vi "auto_alignment-v3.vi"(3 "NM-params":T1={"alpha"=1.0, "gamma"=2.0, "rho"=0.5, "sigma"=0.5, "simplex L"=0.5}) -> (1 "xStart":dbl=264.0 format="%#_13g", 2 "yStart":dbl=123.0 format="%#_13g", 4 "Optimized Location":dbl[](array[numeric]), 8 "std dev of simplex values":dbl, 14 "run time (s)":dbl)   [LabVIEW 2024]
uses:
  <vilib>/Math Plots/3D Math Plots/3D Contour/3D Contour XCtrl/3D Contour.xctl
  208f4aca-97d4-4ce0-8583-53fc1167a3ec.vi
  <vilib>/numeric/Random Number (Range) DBL.vi
  2150a5ec-3bbc-4184-8c90-cd07ede4a1ff.vi
  5b59031f-b1ff-41af-80a7-e72a33ebffa1.vi
  <vilib>/Analysis/baseanly.llb/Real Dot Product.vi
  <vilib>/Array/Sort 2D Array - Pop Stack.vi
  <vilib>/Array/Sort 2D Array - Push Stack.vi
  5b59031f-b1ff-41af-80a7-e72a33ebffa1.vi/269d4b3b-47f5-49e3-8884-44851e4dd9d5.vi
  5b59031f-b1ff-41af-80a7-e72a33ebffa1.vi/6d99389c-673d-4efb-bf33-19b32bcf4cf8.vi
  <vilib>/Utility/file.llb/Read Delimited Spreadsheet (string).vi
  <vilib>/gmath/interp.llb/Create Mesh Grid (2D) (x,y arrays).vi
  <vilib>/Math Plots/3D Math Plots/3D Contour/3D Contour Datatype/Public/Plot Helper (Matrix).vi
  <vilib>/Utility/file.llb/Write Delimited Spreadsheet (DBL).vi
  <vilib>/Analysis/NI_AALBase.lvlib
  O:/DSG/Tyler/EIC/DIRC/daq/automated/Thorlabs.MotionControl.IntegratedStepperMotorsCLI.dll
  Thorlabs.MotionControl.IntegratedStepperMotorsCLI.dll
  <vilib>/Analysis/NI_AALPro.lvlib
  <vilib>/Math Plots/3D Math Plots/3D Contour/3D Contour Datatype/3D Contour Datatype.lvclass
  <vilib>/gmath/NI_Gmath.lvlib
panel:
  out "3D Contour":refnum<class "3D Plot Datatype.lvclass">[](xcontrol)
  out "z-angle converge":bool
  in  "z-angle-limit":dbl=0.04 caption="Z-Angle Convergence Goal"
  in  "squError-limit":dbl=0.04 caption="Squared Error Convergence Goal"
  out "angle-to-z":dbl
  out "squared error limit":bool
  out "SquError":dbl
  out "x_c":dbl[](array[numeric])
  out "x_e":dbl[](array[numeric])
  out "x_r":dbl[](array[numeric])
  out "x_o":dbl[](array[numeric])
  out "sim-pdx":dbl[](array[numeric])
  out "sim-pdy":dbl[](array[numeric])
  out "sim-iCorr":dbl[](array[numeric])
  out "sim_max":dbl[](array[numeric])
  out "sim_x-range":dbl[](array[numeric])
  out "sim_y-range":dbl[](array[numeric])
  out "termination-test-simplex":dbl[][](array[numeric])
  out "timeout":bool
  out "simplex converge":bool
  out "value converge":bool
  out "simplex leg lengths":dbl[](array[numeric])
  out "nPts tested":dbl
  out "sim-data":dbl[][](array[numeric])
  in  "simplex-limit":dbl=1e-06 caption="Simplex Length Convergence Goal" format="%#_13g"
  in  "value-limit":dbl=1e-06 caption="Value Convergence Goal" format="%#_13g"
  out "Pts Tested":dbl[][](array[numeric])
  in  "stop":bool
  # "Test Sub-Points"
  # "centroid"
  # "reflection point"
  # "expansion point"
  # "contraction point"
  # "Model Data"
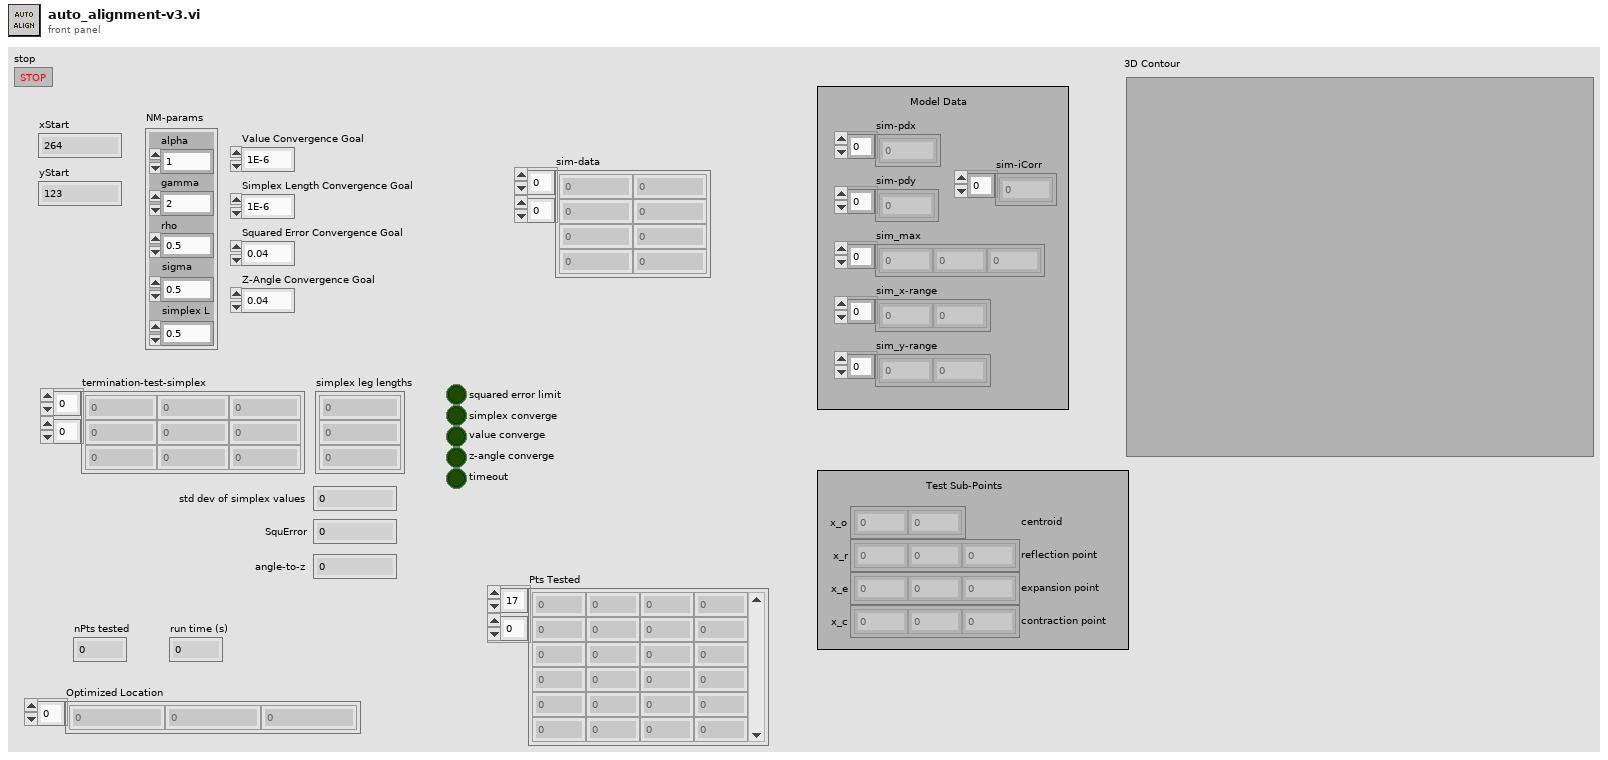
[diagram p1: front panel]
types:
  T1 = cluster{"alpha":dbl, "gamma":dbl, "rho":dbl, "sigma":dbl, "simplex L":dbl}
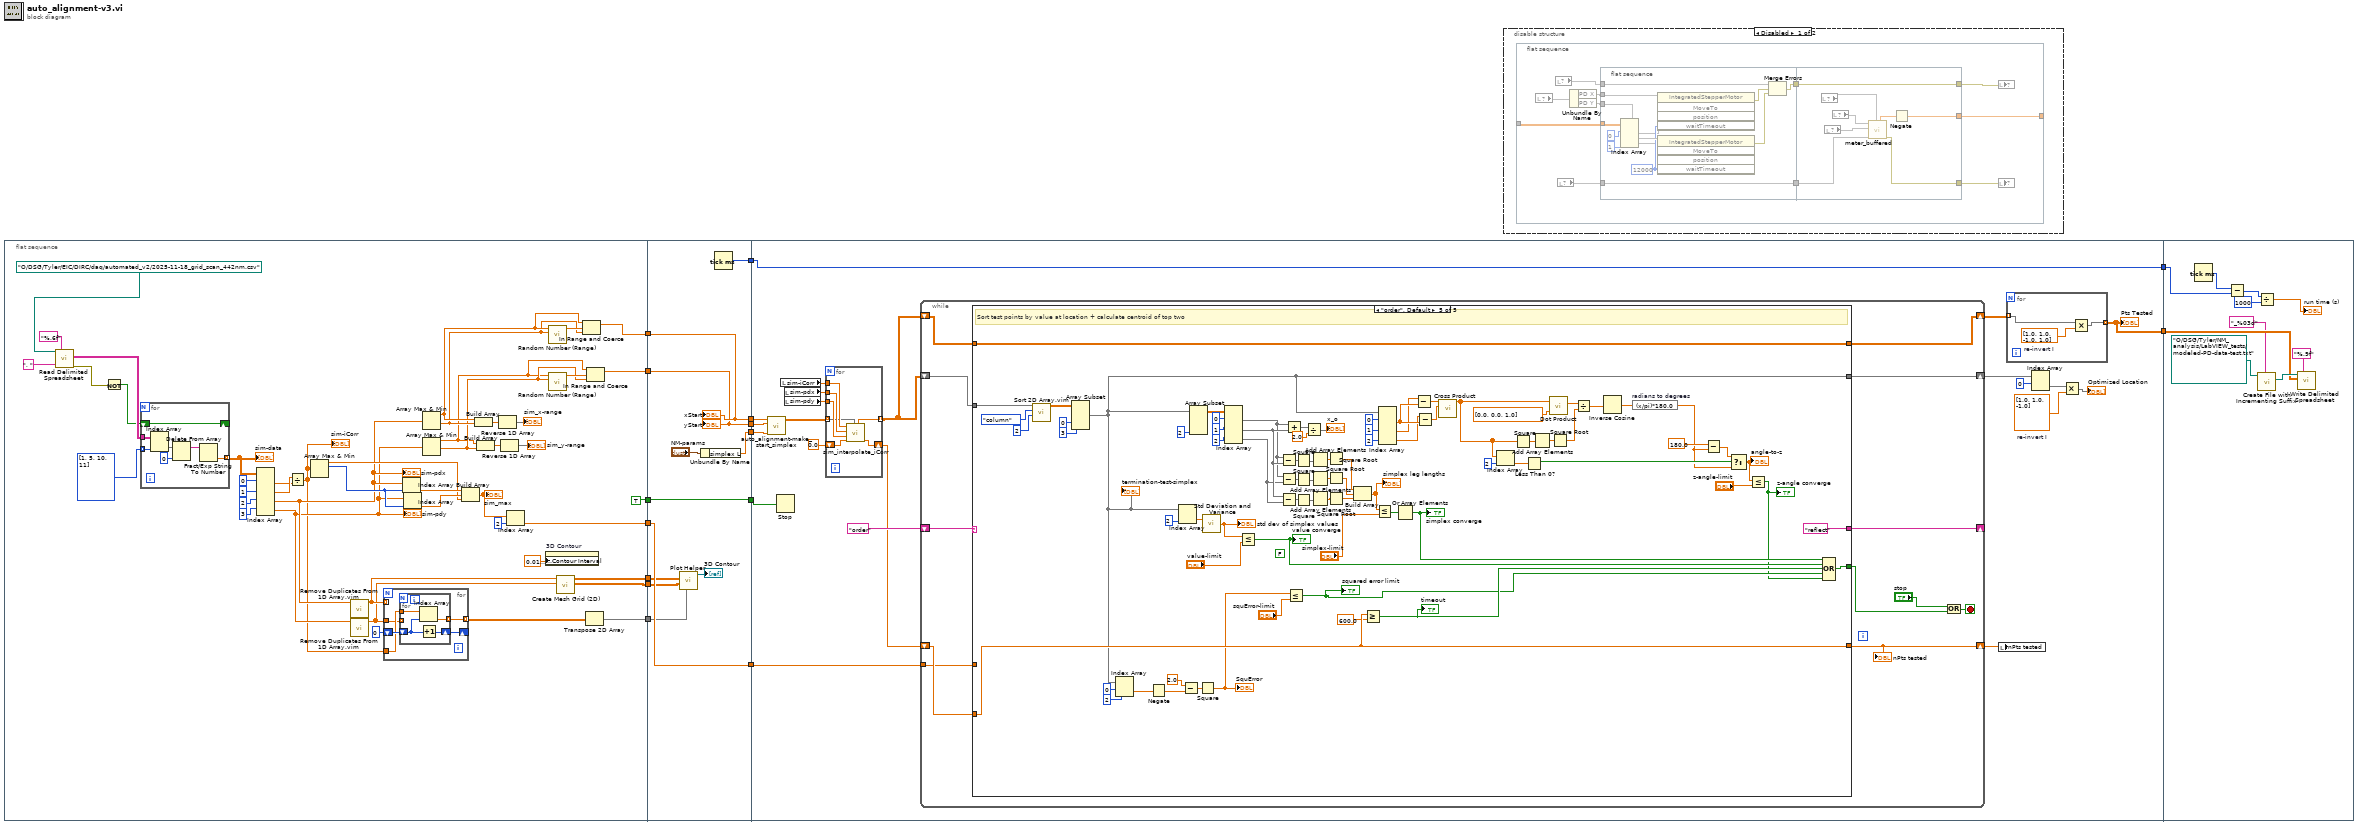
[diagram p0: block diagram]
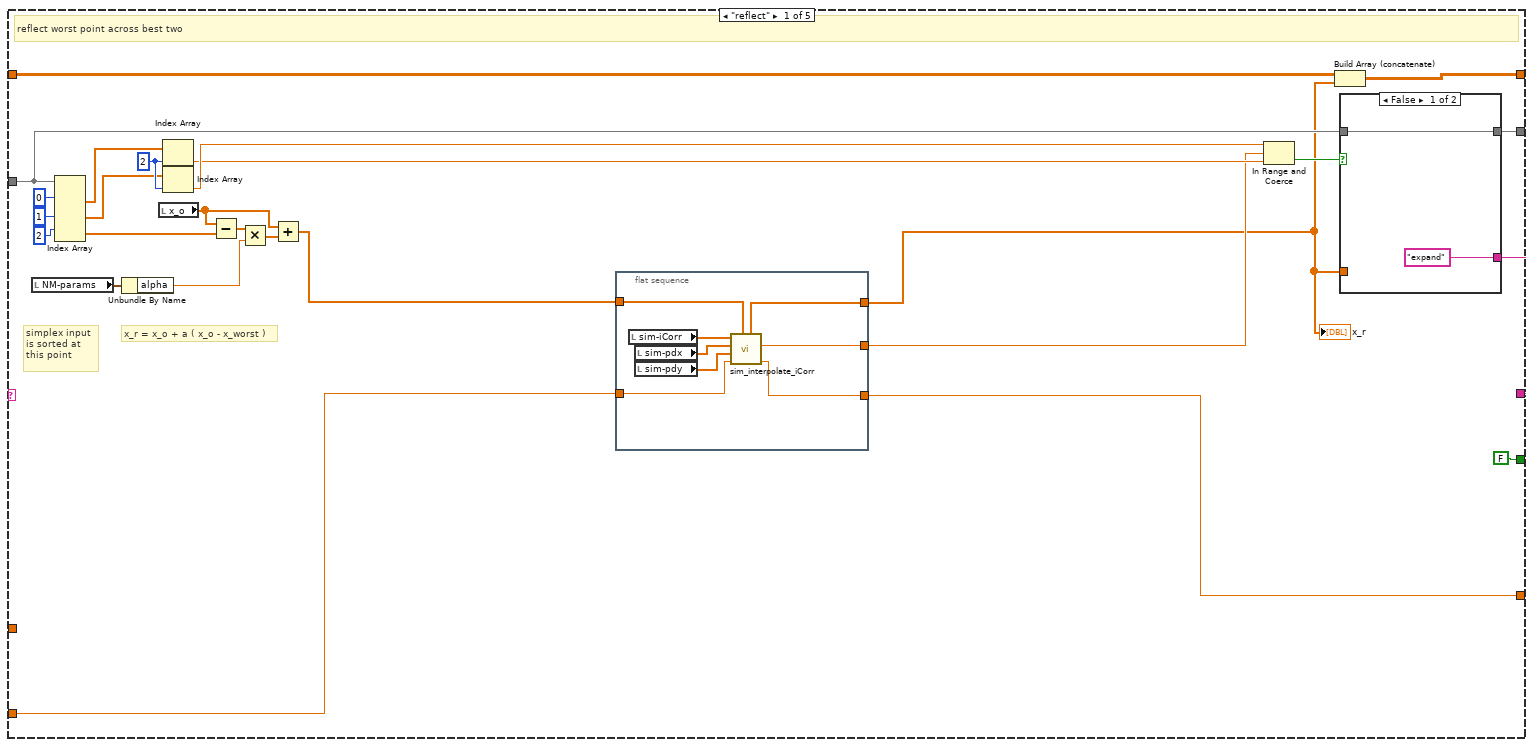
[diagram p3: hidden frame]
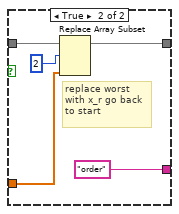
[diagram p4: hidden frame]
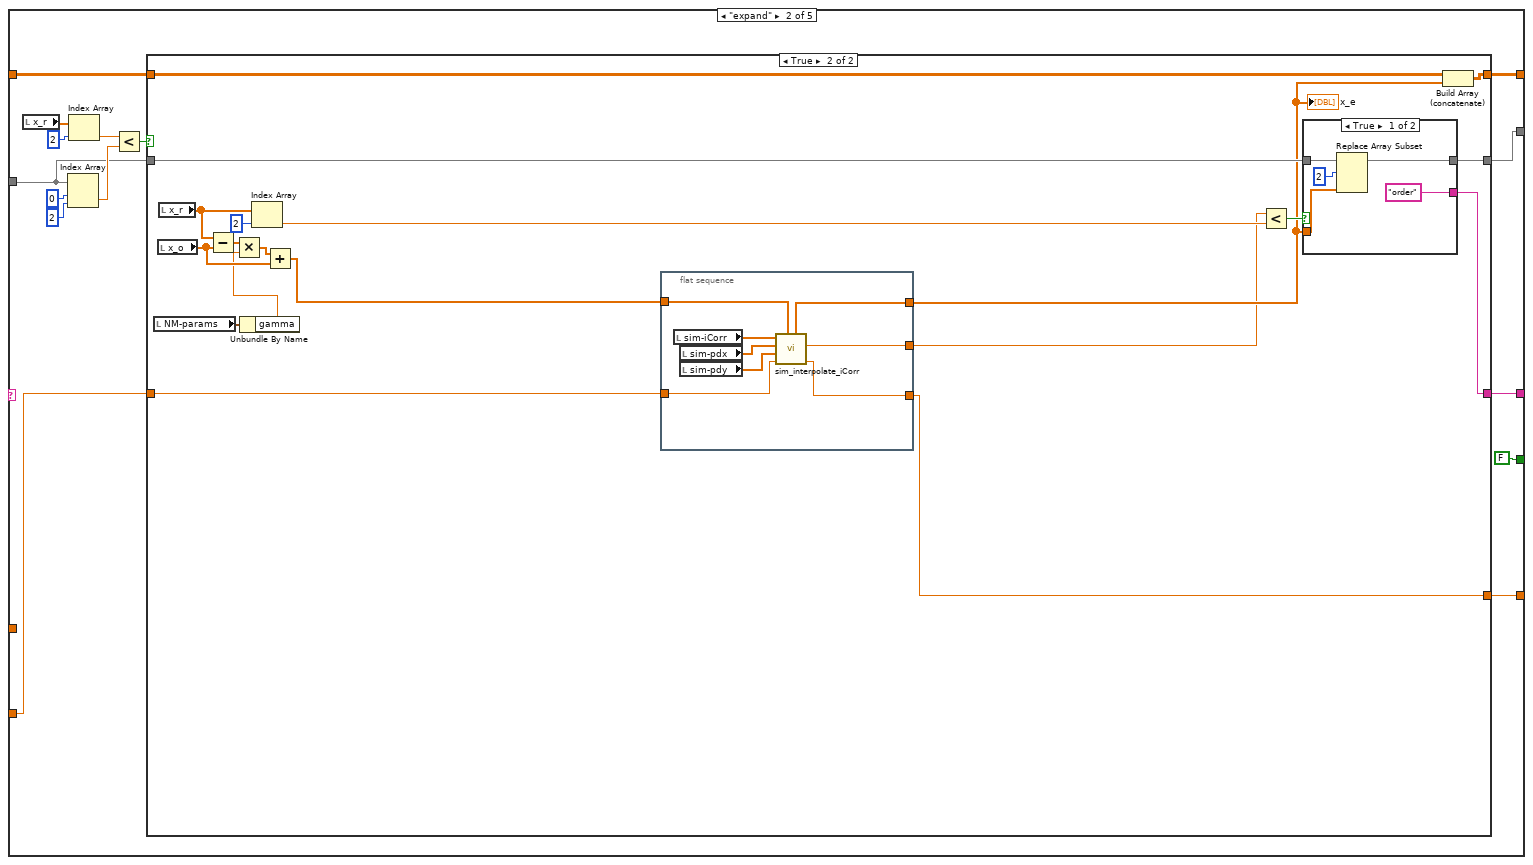
[diagram p5: hidden frame]
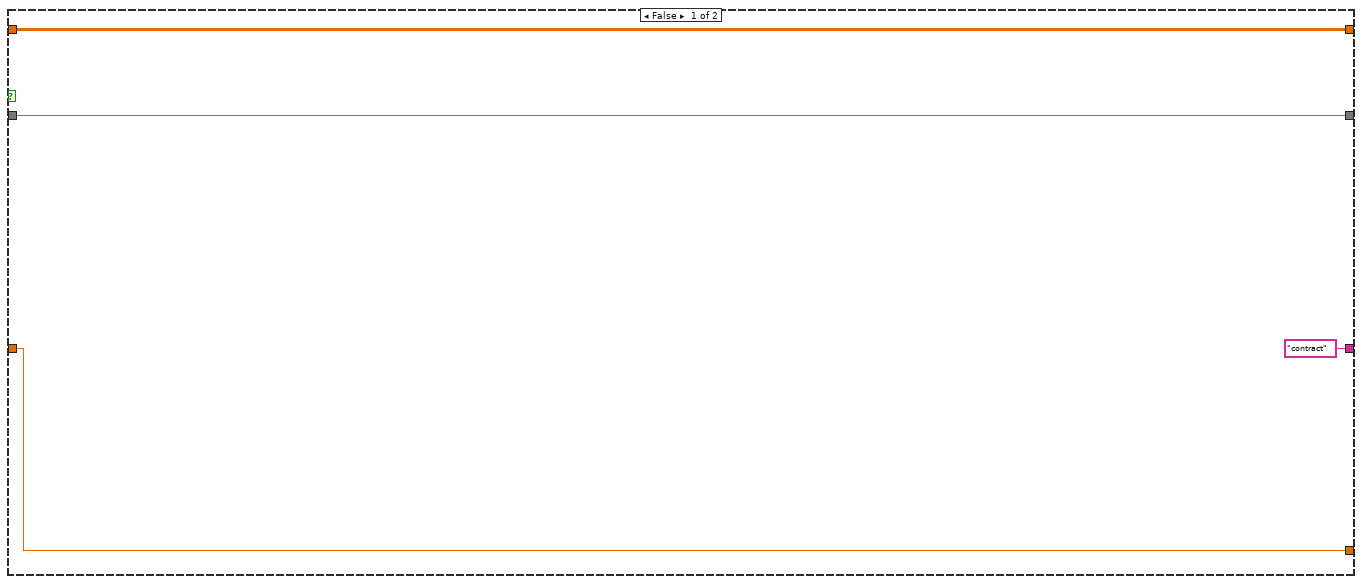
[diagram p6: hidden frame]
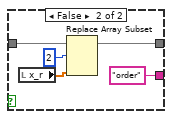
[diagram p7: hidden frame]
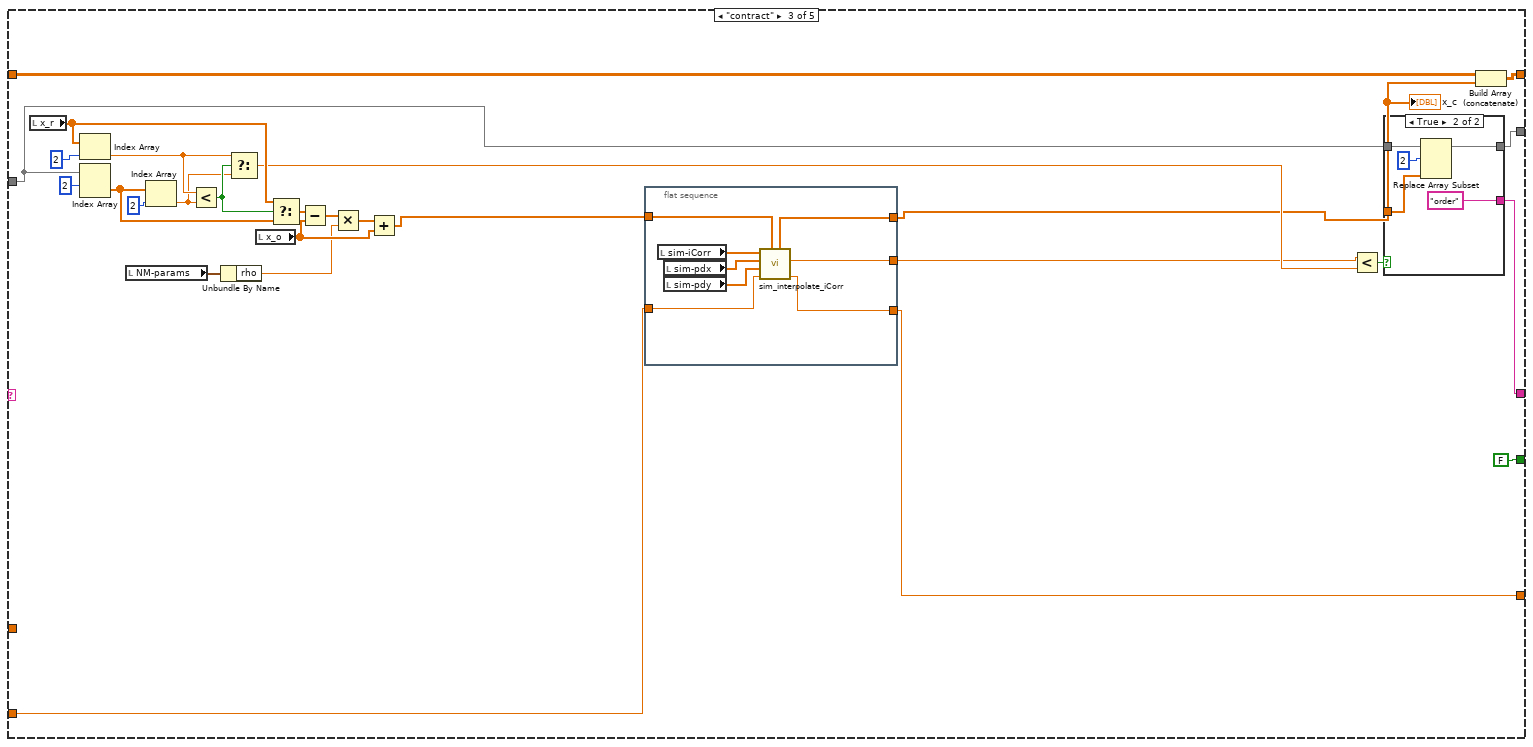
[diagram p8: hidden frame]
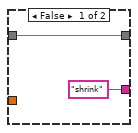
[diagram p9: hidden frame]
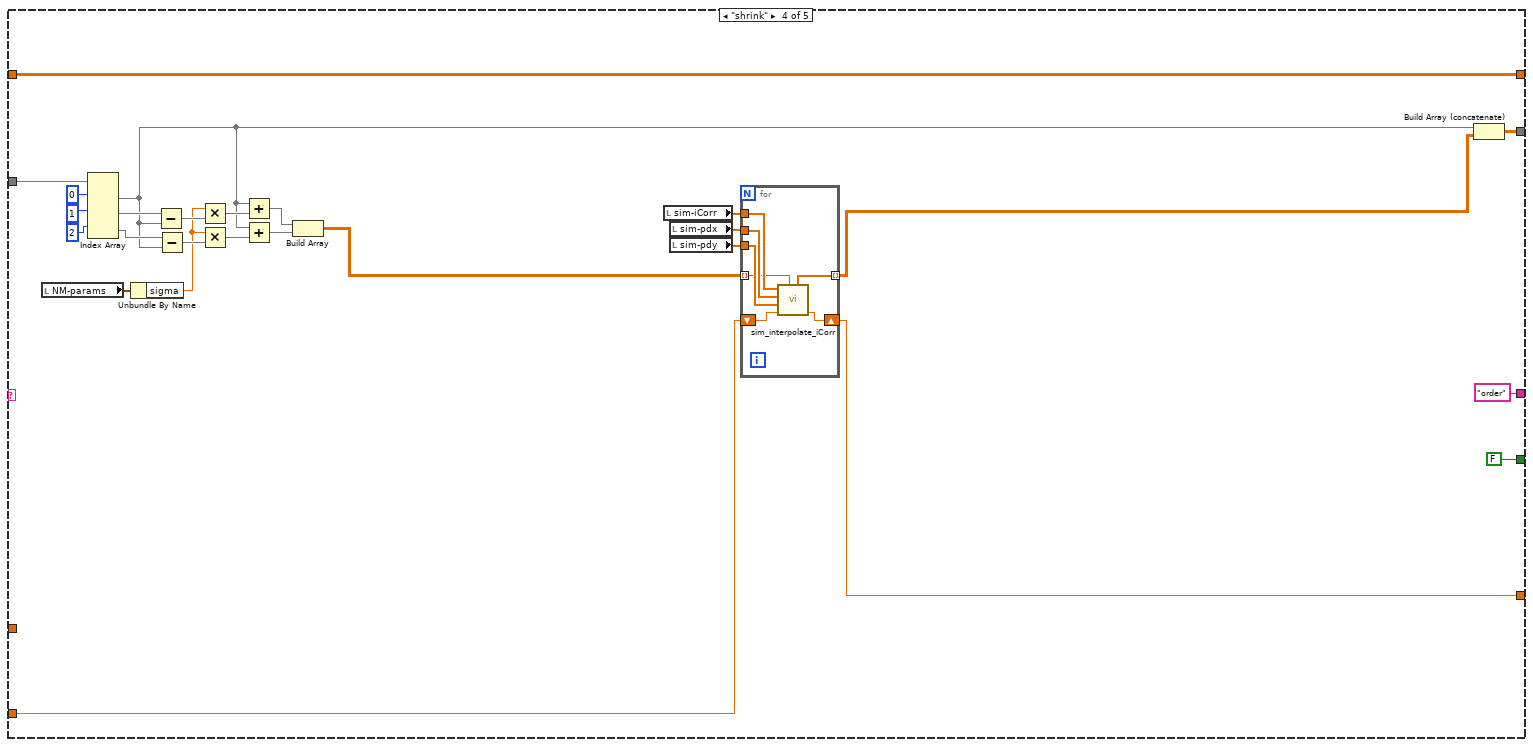
[diagram p10: hidden frame]
diagram:
  n1 = flat-sequence {
    tunnel: [w39] -> w9
    tunnel: [w36] -> w8
    tunnel: [w29] -> w7
    tunnel: [TRUE] -> w5
    tunnel: [w18] -> w3
    tunnel: [w17] -> w2
    tunnel: [w21] -> w1
    tunnel: [w87] -> w15
    tunnel: [w83] -> w13
    tunnel: [w84] -> w12
    tunnel: [w85] -> w11
    tunnel: w9 -> [w84]
    tunnel: w8 -> [w83]
    tunnel: w7 -> [w82]
    tunnel: [w82] -> w6
    tunnel: w5 -> [w81]
    tunnel: [w81] -> w4
    tunnel: w3 -> [w79]
    tunnel: w2 -> [w78]
    tunnel: w1 -> [w77]
    tunnel: w15 -> [w108]
    tunnel: [w108] -> w14
    tunnel: w13 -> [w96]
    tunnel: w12 -> [w97]
    tunnel: w11 -> [w95]
    tunnel: [w90] -> w10
    tunnel: w6 -> [w89]
    tunnel: w4 -> [w88]
    tunnel: w14 -> [w391]
    tunnel: w10 -> [w386]
    frame #0 {
      n2 = call-poly <vilib>:"Read Delimited Spreadsheet.vi"("file path (dialog if empty)"=path "O:/DSG/Tyler/EIC/DIRC/daq/automated_v2/2025-11-18_grid_scan_442nm.csv", "format (%s)"="%.6f" ("format (%.3f)"), "delimiter (\\t)"=", " ("delimiter (\\t)")) -> ("all rows"=w57:string[][], "error out"=w59:errorcluster)  [unwired: 7 in, 4 out]
      n3 = Not(x=w59) -> (.not. x?=w55:bool)
      n4 = for {
        tunnel: i32[] [1, 5, 10, 11] -> [w75] mode=indexing
        tunnel: w57 -> [w76]
        shift-right: [w74] -> _
        shift-left: w55 -> [w74]
        tunnel: [w70] -> w48 mode=indexing
        n5 = Index Array(array=w76, index (col)=w75) -> (element=w73:string[])  [unwired: 1 in]
        n6 = Delete From Array(array=w73, index=0) -> (array with subset deleted=w71:string[])  [unwired: 1 in, 1 out]
        n7 = Fract/Exp String To Number(string=w71) -> (number=w70:dbl[])  [unwired: 3 in, 1 out]
      }
      "sim-data" <- w48
      n8 = Index Array(array=w48, index (row) #1=0 ("index"), index (row) #2=1 ("index (row)"), index (row) #3=2 ("index (row)"), index (row) #4=3 ("index (row)")) -> (element #1=w49:dbl[], element #2=w50:dbl[], element #3=w25:dbl[], element #4=w24:dbl[])  [unwired: 4 in]
      "sim-pdx" <- w25
      "sim-pdy" <- w24
      n9 = Divide(x=w50, y=w49) -> (x/y=w23:dbl[])
      "sim-iCorr" <- w23
      n10 = Array Max & Min(array=w23) -> (max value=w26:dbl, max index (indices)=w47:i32)  [unwired: 2 out]
      n11 = call "Remove Duplicates From 1D Array.vim"("array"=w25) -> ("array with duplicates removed"=w20:dbl[])  [unwired: 10 in]
      n12 = call "Remove Duplicates From 1D Array.vim"("array"=w24) -> ("array with duplicates removed"=w19:dbl[])  [unwired: 10 in]
      n13 = for {
        tunnel: w20 -> [_] mode=indexing
        tunnel: w19 -> [w61]
        tunnel: w23 -> [w62]
        tunnel: [w65] -> w22 mode=indexing
        shift-right: [w63] -> _
        shift-left: 0 -> [w64]
        n14 = for {
          tunnel: [w69] -> w65 mode=indexing
          shift-right: [w68] -> w63
          shift-left: w64 -> [w67]
          tunnel: w62 -> [w66]
          tunnel: w61 -> [_] mode=indexing
          n15 = Index Array(array=w66, index=w67) -> (element=w69:dbl)
          n16 = Increment(x=w67) -> (x+1=w68:i32)
        }
      }
      n17 = Index Array(array=w25, index=w47) -> (element=w46:dbl)
      n18 = Index Array(array=w24, index=w47) -> (element=w45:dbl)
      n19 = Array Max & Min(array=w25) -> (max value=w38:dbl, min value=w37:dbl)  [unwired: 2 out]
      n20 = Array Max & Min(array=w24) -> (max value=w33:dbl, min value=w34:dbl)  [unwired: 2 out]
      n21 = Build Array(w46, w45, w26) -> (w31:dbl[])
      "sim_max" <- w31
      n22 = Build Array(w38, w37) -> (w43:dbl[])
      n23 = Build Array(w33, w34) -> (w44:dbl[])
      n24 = Reverse 1D Array(array=w43) -> (reversed array=→"sim_x-range":dbl[])
      n25 = Reverse 1D Array(array=w44) -> (reversed array=→"sim_y-range":dbl[])
      n26 = Index Array(array=w31, index=2) -> (element=w29:dbl)
      n27 = property on="3D Contour" class="3D Contour (strict)"("Plot Specific:Contour Interval"=sgl 0.02 ("Plot Specific:Contour:Contour Interval")) -> ()  [unwired: 2 in, 2 out]
      n28 = call-poly <vilib>:"Random Number (Range).vi"("lower bound (0)"=w37, "upper bound (100)"=w38) -> ("number"=w40:dbl)  [unwired: 9 in]
      n29 = call-poly <vilib>:"Random Number (Range).vi"("lower bound (0)"=w34, "upper bound (100)"=w33) -> ("number"=w35:dbl)  [unwired: 9 in]
      n30 = call-poly <vilib>:"Create Mesh Grid (2D).vi"("y domain"=w19, "x domain"=w20) -> ("Y"=w17:dbl[][], "X"=w18:dbl[][])  [unwired: 7 in, 1 out]
      n31 = In Range and Coerce(upper limit=w38, x=w40, lower limit=w37) -> (coerced(x)=w39:dbl)  [unwired: 1 out]
      n32 = Transpose 2D Array(2D array=w22) -> (transposed array=w21:dbl[][])
      n33 = In Range and Coerce(upper limit=w33, x=w35, lower limit=w34) -> (coerced(x)=w36:dbl)  [unwired: 1 out]
    }
    frame #1 {
      n34 = call-poly <vilib>:"Plot Helper.vi"("z matrix"=w77, "y matrix"=w78, "x matrix"=w79) -> ("3D Plot lvclass Array out"=→"3D Contour":refnum<class "3D Plot Datatype.lvclass">[])  [unwired: 3 in, 5 out]
      n35 = Unbundle By Name("NM-params") -> ("simplex L"=w85:dbl)
      n36 = Tick Count (ms)() -> (millisecond timer value=w87:u32)
      "xStart" <- w84
      "yStart" <- w83
    }
    frame #2 {
      w103 = dbl[] [1.0, 1.0, -1.0]  # re-invert I
      n37 = call "auto_alignment-make_start_simplex.vi"("L"=w95, "yStart"=w96, "xStart"=w97) -> ("Array"=w98:dbl[][])  [unwired: 8 in]
      n38 = Stop(stop? (T)=w88) -> ()
      n39 = local read "sim-iCorr"() -> (w100:dbl[])
      n40 = local read "sim-pdx"() -> (w102:dbl[])
      n41 = local read "sim-pdy"() -> (w101:dbl[])
      n42 = for {
        shift-right: [w114] -> w93
        shift-left: 0.0 -> [w113]
        tunnel: w98 -> [w116] mode=indexing
        tunnel: [w115] -> w94 mode=indexing
        tunnel: w100 -> [w119]
        tunnel: w101 -> [w117]
        tunnel: w102 -> [w118]
        n43 = call "sim_interpolate_iCorr.vi"("point in"=w116, "nPts in"=w113, "sim-pdy"=w117, "sim-pdx"=w118, "sim-iCorr"=w119) -> ("nPts out"=w114:dbl, "measured-point out"=w115:dbl[])  [unwired: 4 in, 1 out]
      }
      n44 = while {
        shift-right: [w129] -> w107
        shift-left: w94 -> [w128]
        shift-right: [w130] -> _
        shift-left: "order" -> [w131]
        shift-right: [w126] -> w91
        shift-left: w94 -> [w127]
        shift-right: [w121] -> w92
        shift-left: w93 -> [w122]
        tunnel: w89 -> [w120]
        stop <- w123 stop-if-true
        n45 = case shown="\"order\", Default" w131 {
          tunnel: w128 -> [w143 w180 w242 w295 w348]
          tunnel: [FALSE FALSE FALSE FALSE w355] -> w125
          tunnel: [w142 w179 w243 w284 w326] -> w129
          tunnel: [w144 w178 w244 "order" "reflect"] -> w130
          tunnel: w127 -> [w140 w176 w238 w282 w352]
          tunnel: [w139 w175 w237 w282 w352] -> w126
          tunnel: w122 -> [w135 w174 w230 w274 w346]
          tunnel: [w134 w173 w229 w273 w346] -> w121
          tunnel: w120 -> [_ _ _ _ _]
          frame "reflect" {
            w151 = 2 ("index")
            # "simplex input\nis sorted at\nthis point"
            # "x_r = x_o + a ( x_o - x_worst )"
            # "reflect worst point across best two"
            n46 = local read "NM-params"() -> (w138:T1)
            n47 = Index Array(array=w143, index (row) #1=0 ("index (row)"), index (row) #2=1 ("index (row)"), index (row) #3=2 ("index (row)")) -> (element #1=w150:dbl[], element #2=w149:dbl[], element #3=w152:dbl[])  [unwired: 3 in]
            n48 = Unbundle By Name(w138) -> ("alpha"=w137:dbl)
            n49 = local read "x_o"() -> (w145:dbl[])
            n50 = Index Array(array=w150, index=w151) -> (element=w147:dbl)
            n51 = Index Array(array=w149, index=w151) -> (element=w148:dbl)
            n52 = Subtract(x=w145, y=w152) -> (x-y=w156:dbl[])
            n53 = Multiply(x=w156, y=w137) -> (x*y=w155:dbl[])
            n54 = Add(x=w145, y=w155) -> (x+y=w133:dbl[])
            n55 = flat-sequence {
              tunnel: w133 -> [w162]
              tunnel: w135 -> [w161]
              tunnel: [w160] -> w134
              tunnel: [w159] -> w132
              tunnel: [w158] -> w136
              frame #0 {
                n56 = local read "sim-iCorr"() -> (w163:dbl[])
                n57 = local read "sim-pdx"() -> (w164:dbl[])
                n58 = local read "sim-pdy"() -> (w165:dbl[])
                n59 = call "sim_interpolate_iCorr.vi"("point in"=w162, "nPts in"=w161, "sim-pdy"=w165, "sim-pdx"=w164, "sim-iCorr"=w163) -> ("nPts out"=w160:dbl, "iCorr out"=w158:dbl, "measured-point out"=w159:dbl[])  [unwired: 4 in]
              }
            }
            n60 = In Range and Coerce(upper limit=w148, x=w136, lower limit=w147) -> (In Range?=w146:bool)  [unwired: 1 out]
            n61 = Build Array (concatenate)(w140, w132) -> (w139:dbl[][])
            n62 = case shown="False" w146 {
              tunnel: ["expand" "order"] -> w144
              tunnel: w143 -> [w166 w172]
              tunnel: [w166 w169] -> w142
              tunnel: w132 -> [_ w170]
              frame False {
              }
              frame True {
                # "replace worst \nwith x_r go back\nto start"
                n63 = Replace Array Subset(array=w172, new element=w170, index (row)=2) -> (w169:dbl[][])  [unwired: 1 in]
              }
            }
            "x_r" <- w132
          }
          frame "expand" {
            n64 = local read "x_r"() -> (w185:dbl[])
            n65 = Index Array(array=w180, index (row)=0, index (col)=2 ("disabled index (col)")) -> (element=w183:dbl)
            n66 = Index Array(array=w185, index=2) -> (element=w182:dbl)
            n67 = Less?(x=w182, y=w183) -> (x < y?=w181:bool)
            n68 = case shown="True" w181 {
              tunnel: w180 -> [w191 w203]
              tunnel: [w191 w202] -> w179
              tunnel: ["contract" w201] -> w178
              tunnel: w176 -> [w189 w200]
              tunnel: [w189 w199] -> w175
              tunnel: w174 -> [w188 w193]
              tunnel: [w188 w192] -> w173
              frame False {
              }
              frame True {
                n69 = local read "NM-params"() -> (w198:T1)
                n70 = local read "x_o"() -> (w208:dbl[])
                n71 = local read "x_r"() -> (w207:dbl[])
                n72 = Subtract(x=w207, y=w208) -> (x-y=w210:dbl[])
                n73 = Unbundle By Name(w198) -> ("gamma"=w197:dbl)
                n74 = Multiply(x=w210, y=w197) -> (x*y=w209:dbl[])
                n75 = Index Array(array=w207, index=2) -> (element=w205:dbl)
                n76 = Add(x=w209, y=w208) -> (x+y=w194:dbl[])
                n77 = flat-sequence {
                  tunnel: w194 -> [w215]
                  tunnel: w193 -> [w214]
                  tunnel: [w213] -> w192
                  tunnel: [w212] -> w196
                  tunnel: [w211] -> w195
                  frame #0 {
                    n78 = local read "sim-iCorr"() -> (w216:dbl[])
                    n79 = local read "sim-pdx"() -> (w217:dbl[])
                    n80 = local read "sim-pdy"() -> (w218:dbl[])
                    n81 = call "sim_interpolate_iCorr.vi"("point in"=w215, "nPts in"=w214, "sim-pdy"=w218, "sim-pdx"=w217, "sim-iCorr"=w216) -> ("nPts out"=w213:dbl, "iCorr out"=w211:dbl, "measured-point out"=w212:dbl[])  [unwired: 4 in]
                  }
                }
                n82 = Less?(x=w195, y=w205) -> (x < y?=w204:bool)
                n83 = case shown="True" w204 {
                  tunnel: w203 -> [w222 w227]
                  tunnel: w196 -> [w221 _]
                  tunnel: [w220 w226] -> w202
                  tunnel: ["order" "order"] -> w201
                  frame True {
                    n84 = Replace Array Subset(array=w222, new element=w221, index (row)=2) -> (w220:dbl[][])  [unwired: 1 in]
                  }
                  frame False {
                    n85 = local read "x_r"() -> (w224:dbl[])
                    n86 = Replace Array Subset(array=w227, new element=w224, index (row)=2) -> (w226:dbl[][])  [unwired: 1 in]
                  }
                }
                n87 = Build Array (concatenate)(w200, w196) -> (w199:dbl[][])
                "x_e" <- w196
              }
            }
          }
          frame "contract" {
            n88 = local read "x_r"() -> (w252:dbl[])
            n89 = Index Array(array=w252, index=2) -> (element=w247:dbl)
            n90 = Index Array(array=w242, index (row)=2) -> (element=w251:dbl[])  [unwired: 1 in]
            n91 = local read "NM-params"() -> (w236:T1)
            n92 = Index Array(array=w251, index=2) -> (element=w246:dbl)
            n93 = Less?(x=w247, y=w246) -> (x < y?=w248:bool)
            n94 = Unbundle By Name(w236) -> ("rho"=w235:dbl)
            n95 = Select(t=w247, s=w248, f=w246) -> (s? t:f=w234:dbl)
            n96 = local read "x_o"() -> (w240:dbl[])
            n97 = Select(t=w252, s=w248, f=w251) -> (s? t:f=w250:dbl[])
            n98 = Subtract(x=w250, y=w240) -> (x-y=w249:dbl[])
            n99 = Multiply(x=w249, y=w235) -> (x*y=w241:dbl[])
            n100 = Add(x=w241, y=w240) -> (x+y=w232:dbl[])
            n101 = flat-sequence {
              tunnel: w232 -> [w260]
              tunnel: w230 -> [w259]
              tunnel: [w258] -> w229
              tunnel: [w257] -> w231
              tunnel: [w256] -> w233
              frame #0 {
                n102 = local read "sim-iCorr"() -> (w261:dbl[])
                n103 = local read "sim-pdx"() -> (w262:dbl[])
                n104 = local read "sim-pdy"() -> (w263:dbl[])
                n105 = call "sim_interpolate_iCorr.vi"("point in"=w260, "nPts in"=w259, "sim-pdy"=w263, "sim-pdx"=w262, "sim-iCorr"=w261) -> ("nPts out"=w258:dbl, "iCorr out"=w256:dbl, "measured-point out"=w257:dbl[])  [unwired: 4 in]
              }
            }
            n106 = Less?(x=w233, y=w234) -> (x < y?=w245:bool)
            n107 = case shown="True" w245 {
              tunnel: ["shrink" "order"] -> w244
              tunnel: [w264 w266] -> w243
              tunnel: w242 -> [w264 w268]
              tunnel: w231 -> [_ w267]
              frame False {
              }
              frame True {
                n108 = Replace Array Subset(array=w268, new element=w267, index (row)=2) -> (w266:dbl[][])  [unwired: 1 in]
              }
            }
            n109 = Build Array (concatenate)(w238, w231) -> (w237:dbl[][])
            "x_c" <- w231
          }
          frame "shrink" {
            n110 = local read "NM-params"() -> (w279:T1)
            n111 = Index Array(array=w295, index (row) #1=0 ("index (row)"), index (row) #2=1 ("index (row)"), index (row) #3=2 ("index (row)")) -> (element #1=w285:dbl[], element #2=w291:dbl[], element #3=w290:dbl[])  [unwired: 3 in]
            n112 = Unbundle By Name(w279) -> ("sigma"=w278:dbl)
            n113 = Subtract(x=w291, y=w285) -> (x-y=w288:dbl[])
            n114 = Subtract(x=w290, y=w285) -> (x-y=w289:dbl[])
            n115 = Multiply(x=w278, y=w288) -> (x*y=w287:dbl[])
            n116 = Multiply(x=w278, y=w289) -> (x*y=w286:dbl[])
            n117 = Add(x=w285, y=w287) -> (x+y=w281:dbl[])
            n118 = Add(x=w285, y=w286) -> (x+y=w280:dbl[])
            n119 = Build Array(w281, w280) -> (w271:dbl[][])
            n120 = local read "sim-iCorr"() -> (w275:dbl[])
            n121 = local read "sim-pdx"() -> (w277:dbl[])
            n122 = local read "sim-pdy"() -> (w276:dbl[])
            n123 = for {
              shift-right: [w298] -> w273
              shift-left: w274 -> [w297]
              tunnel: w271 -> [w300] mode=indexing
              tunnel: [w299] -> w272 mode=indexing
              tunnel: w275 -> [w303]
              tunnel: w276 -> [w301]
              tunnel: w277 -> [w302]
              n124 = call "sim_interpolate_iCorr.vi"("point in"=w300, "nPts in"=w297, "sim-pdy"=w301, "sim-pdx"=w302, "sim-iCorr"=w303) -> ("nPts out"=w298:dbl, "measured-point out"=w299:dbl[])  [unwired: 4 in, 1 out]
            }
            n125 = Build Array (concatenate)(w285, w272) -> (w284:dbl[][])
          }
          frame "order", Default {
            (unwired) FALSE
            # "Sort test points by value at location + calculate centroid of top two"
            n126 = call "Sort 2D Array.vim"("index"=2, "dimension to index (column)"=enum16{"column", "row"}."column", "2D array"=w348) -> ("sorted 2D array"=w347:dbl[][])  [unwired: 7 in, 1 out]
            n127 = Array Subset(array=w347, index (col)=0 ("index"), length (col)=3 ("length")) -> (w326:dbl[][])  [unwired: 2 in]
            "termination-test-simplex" <- w326
            n128 = Index Array(array=w326, index (row)=0, index (col)=2 ("disabled index (col)")) -> (element=w341:dbl)
            n129 = Negate(x=w341) -> (-x=w339:dbl)
            n130 = Index Array(array=w326, index (col)=2 ("index")) -> (element=w372:dbl[])  [unwired: 1 in]
            n131 = Subtract(x=2.0, y=w339) -> (x-y=w340:dbl)
            n132 = Array Subset(array=w326, length (col)=2 ("length")) -> (w371:dbl[][])  [unwired: 3 in]
            n133 = Square(x=w340) -> (x^2=w338:dbl)
            "SquError" <- w338
            n134 = call <vilib>:"Std Deviation and Variance.vi"("X"=w372) -> ("standard deviation"=w353:dbl)  [unwired: 1 in, 2 out]
            "std dev of simplex values" <- w353
            n135 = Index Array(array=w371, index (row) #1=0 ("index (row)"), index (row) #2=1 ("index (row)"), index (row) #3=2 ("index (row)")) -> (element #1=w336:dbl[], element #2=w337:dbl[], element #3=w335:dbl[])  [unwired: 3 in]
            n136 = Less Or Equal?(x=w353, y="value-limit") -> (x <= y?=w310:bool)
            "value converge" <- w310
            n137 = Subtract(x=w336, y=w337) -> (x-y=w369:dbl[])
            n138 = Subtract(x=w336, y=w335) -> (x-y=w361:dbl[])
            n139 = Subtract(x=w337, y=w335) -> (x-y=w364:dbl[])
            n140 = Add(x=w336, y=w337) -> (x+y=w376:dbl[])
            n141 = Less Or Equal?(x=w338, y="squError-limit") -> (x <= y?=w305:bool)
            "squared error limit" <- w305
            n142 = Square(x=w369) -> (x^2=w368:dbl[])
            n143 = Square(x=w361) -> (x^2=w365:dbl[])
            n144 = Square(x=w364) -> (x^2=w363:dbl[])
            n145 = Divide(x=w376, y=2.0) -> (x/y=→"x_o":dbl[])
            n146 = Add Array Elements(numeric array=w368) -> (sum=w367:dbl)
            n147 = Add Array Elements(numeric array=w365) -> (sum=w366:dbl)
            n148 = Add Array Elements(numeric array=w363) -> (sum=w362:dbl)
            n149 = Square Root(x=w367) -> (sqrt(x)=w358:dbl)
            n150 = Square Root(x=w366) -> (sqrt(x)=w359:dbl)
            n151 = Square Root(x=w362) -> (sqrt(x)=w360:dbl)
            n152 = Build Array(w358, w359, w360) -> (w357:dbl[])
            "simplex leg lengths" <- w357
            n153 = Greater Or Equal?(x=w346, y=600.0) -> (x >= y?=w344:bool)
            "timeout" <- w344
            n154 = Less Or Equal?(x=w357, y="simplex-limit") -> (x <= y?=w356:bool[])
            n155 = Index Array(array=w326, index (row) #1=0 ("index (row)"), index (row) #2=1 ("index (row)"), index (row) #3=2 ("index (row)")) -> (element #1=w322:dbl[], element #2=w321:dbl[], element #3=w320:dbl[])  [unwired: 3 in]
            n156 = Or Array Elements(Boolean array=w356) -> (logical OR=w354:bool)
            "simplex converge" <- w354
            n157 = Subtract(x=w321, y=w322) -> (x-y=w334:dbl[])
            n158 = Subtract(x=w320, y=w322) -> (x-y=w333:dbl[])
            n159 = call <vilib>:"Cross Product.vi"("B Vector"=w333, "A Vector"=w334) -> ("Cross Product"=w318:dbl[])  [unwired: 8 in, 1 out]
            n160 = Index Array(array=w318, index=2) -> (element=w316:dbl)
            n161 = Square(x=w318) -> (x^2=w332:dbl[])
            n162 = Less Than 0?(x=w316) -> (x < 0?=w315:bool)
            n163 = Add Array Elements(numeric array=w332) -> (sum=w331:dbl)
            n164 = call-poly <vilib>:"Dot Product.vi"("Y Vector"=dbl[] [0.0, 0.0, 1.0], "X Vector"=w318) -> ("X * Y"=w329:dbl)  [unwired: 1 out]
            n165 = Square Root(x=w331) -> (sqrt(x)=w328:dbl)
            n166 = Divide(x=w329, y=w328) -> (x/y=w319:dbl)
            n167 = Inverse Cosine(1:w319) -> (0:w327:dbl)
            n168 = expression code="(x/pi)*180.0" "radians to degrees"(w327) -> (w312:dbl)
            n169 = Subtract(x=180.0, y=w312) -> (x-y=w314:dbl)
            n170 = Select(t=w314, s=w315, f=w312) -> (s? t:f=w311:dbl)
            "angle-to-z" <- w311
            n171 = Less Or Equal?(x=w311, y="z-angle-limit") -> (x <= y?=w304:bool)
            "z-angle converge" <- w304
            n172 = Compound Arithmetic op=OR(w354, w310, w344, w305, w304) -> (w355:bool)
          }
        }
        "nPts tested" <- w121
        n173 = Compound Arithmetic op=OR("stop", w125) -> (w123:bool)
      }
      n174 = local write "nPts tested"(w92) -> ()
      n175 = for {
        tunnel: [w111] -> w90 mode=indexing
        tunnel: w91 -> [w112] mode=indexing
        w110 = dbl[] [1.0, 1.0, -1.0, 1.0]  # re-invert I
        n176 = Multiply(x=w112, y=w110) -> (x*y=w111:dbl[])
      }
      "Pts Tested" <- w90
      n177 = Index Array(array=w107, index (row)=0) -> (element=w104:dbl[])  [unwired: 1 in]
      n178 = Multiply(x=w104, y=w103) -> (x*y=→"Optimized Location":dbl[])
    }
    frame #3 {
      n179 = Tick Count (ms)() -> (millisecond timer value=w392:u32)
      n180 = Subtract(x=w392, y=w391) -> (x-y=w390:u32)
      n181 = Divide(x=w390, y=u32 1000) -> (x/y=→"run time (s)":dbl)
      n182 = call <vilib>:"Create File with Incrementing Suffix.vi"("format string (\" (%d)\")"="_%03d" ("format string (\" (%d)\")"), "file path"=path "O:/DSG/Tyler/NM_analysis/LabVIEW_tests/modeled-PD-data-test.txt" ("file path (dialog if empty)")) -> ("actual path"=w387:path)  [unwired: 7 in, 2 out]
      n183 = call-poly <vilib>:"Write Delimited Spreadsheet.vi"("file path (dialog if empty)"=w387, "format (%.3f)"="%.9f", "2D data"=w386) -> ()  [unwired: 11 in, 2 out]
    }
  }
  n184 = disable-structure shown="Disabled" {
    frame Disabled {
      n185 = flat-sequence {
        tunnel: [w401] -> _
        tunnel: [w393] -> _
        frame #0 {
          n186 = local read item#-1() -> (w397)
          n187 = local read item#-1() -> (w398)
          n188 = local read item#-1() -> (w396)
          n189 = Unbundle By Name(w397) -> ("PD X"=w403, "PD Y"=w402)
          n190 = flat-sequence {
            tunnel: w403 -> [w414]
            tunnel: w402 -> [w413]
            tunnel: w398 -> [w407]
            tunnel: [w405] -> w393
            tunnel: w396 -> [w404]
            tunnel: [w406] -> w395
            tunnel: [w404] -> w394
            tunnel: [w424] -> w399
            tunnel: [w421] -> w400
            tunnel: [w417] -> w401
            tunnel: w395 -> [w424]
            tunnel: w394 -> [w422]
            frame #0 {
              w412 = 12000 ("waitTimeout")
              n191 = Index Array(array=w405, index (row) #1=0 ("index"), index (row) #2=1 ("index")) -> (element #1=w409, element #2=w408)  [unwired: 2 in]
              n192 = invoke class="IntegratedStepperMotor" method="MoveTo"(reference=w414, "position"=w409, "waitTimeout"=w412) -> (error out=w416:errorcluster)  [unwired: 2 in, 4 out]
              n193 = invoke class="IntegratedStepperMotor" method="MoveTo"(reference=w413, "position"=w408, "waitTimeout"=w412) -> (error out=w415:errorcluster)  [unwired: 2 in, 4 out]
              n194 = Merge Errors(w407, w416, w415) -> (w406:errorcluster)
            }
            frame #1 {
              n195 = local read item#-1() -> (w420)
              n196 = local read item#-1() -> (w418)
              n197 = local read item#-1() -> (w419)
              n198 = call "meter_buffered.vi"("Samples"=w420, "error in"=w422, "PD ranges"=w418, "meter-VISA"=w419) -> ("error out"=w421:errorcluster, "iCorr"=w423:dbl)  [unwired: 3 in, 3 out]
              n199 = Negate(x=w423) -> (-x=w417:dbl)
            }
          }
          n200 = local write item#-1(w399) -> ()
          n201 = local write item#-1(w400) -> ()
        }
      }
    }
    frame Enabled {
    }
  }
